vi "Shutdown.vi"(11 "Sound Visualizer in":refnum<class "Sound Visualizer.lvclass">) -> (0 "error out":errorcluster, 3 "Sound Visualizer out":refnum<class "Sound Visualizer.lvclass">)   [LabVIEW 2017, in "Sound Visualizer.lvclass"]
uses:
  Sound Visualizer.lvclass
  Sound Visualizer.lvclass/Sound Visualizer.ctl
  Visualizer/Visualizer Type ID.ctl
  Visualizer/Visualizer.lvlib
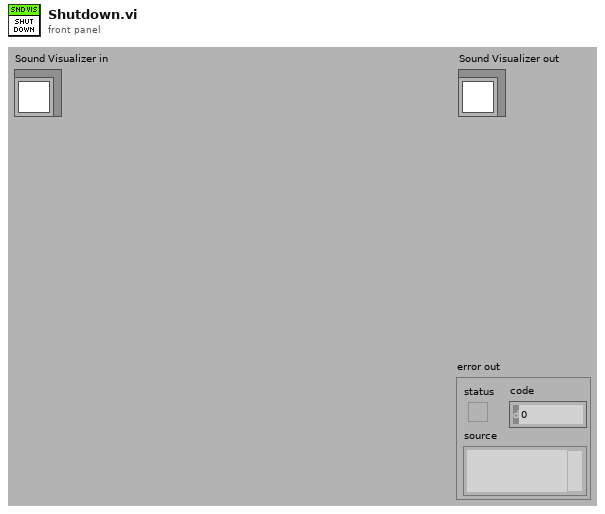
[diagram p1: front panel]
types:
  T1 = typedef "Visualizer.lvlib/Visualizer Type ID.ctl" = u32
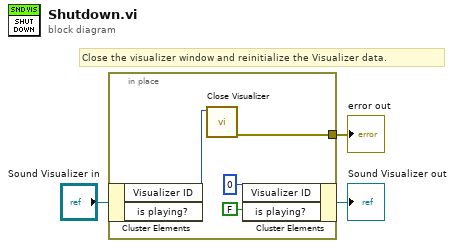
[diagram p0: block diagram]
diagram:
  # "Close the visualizer window and reinitialize the Visualizer data."
  n1 = in-place {
    in-place-border: [w6] -> w1
    n2 = in-place-cluster #1("Sound Visualizer in") -> ("Visualizer ID"=w7:T1)  [unwired: 1 out]
    n3 = call "Close Visualizer.vi"("Visualizer ID"=w7) -> ("error out"=w6:errorcluster)  [unwired: 10 in]
    n4 = in-place-cluster #1("Visualizer ID"=T1 0, "is playing?"=FALSE) -> (→"Sound Visualizer out":refnum<class "Sound Visualizer.lvclass">)
  }
  "error out" <- w1
